vi "reprGraphical.vi"(8 "error in (no error)":errorcluster, 9 "Image Descriptor":T1={"Upper-Left Corner Coordinates"={"UTM Zone"=0, "Hemisphere"=enum."North", "East"=0.0, "North"=0.0}, "Meters/Pixel"=42.294203} {"Upper-Left Corner Coordinates"."North" format="%#_10f"; "Upper-Left Corner Coordinates"."East" format="%#_8f"}, 10 "Image In":T3, 11 "GenericMission in":refnum<class "GenericMission.lvclass">) -> (0 "error out":errorcluster, 2 "Image Out":T3, 3 "GenericMission out":refnum<class "GenericMission.lvclass">)   [LabVIEW 2011, in "GenericMission.lvclass"]
uses:
  GenericMission.lvclass
  <vilib>/vision/Image Controls.llb/IMAQ Image.ctl
  0-OCU/0 Code/mission input/0-Image Descriptor.ctl
  2 Typedefs/UTM Location.ctl
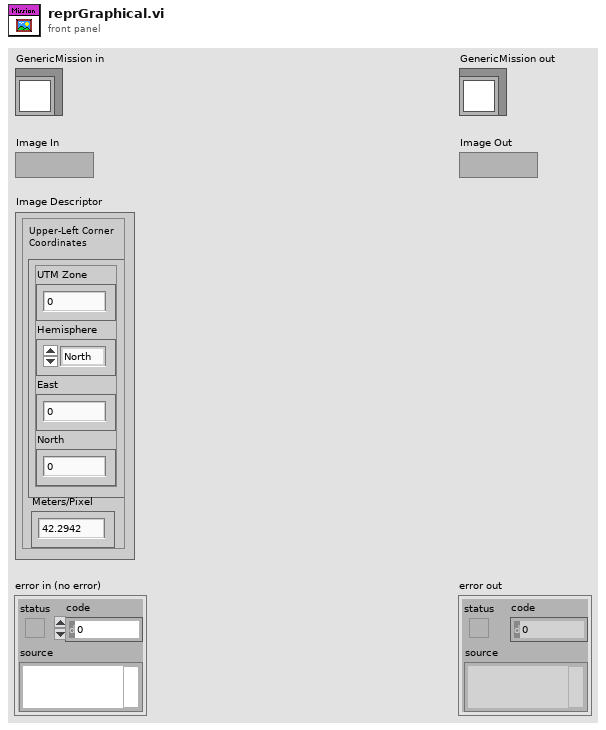
[diagram p1: front panel]
types:
  T1 = typedef "0-Image Descriptor.ctl" = cluster{"Upper-Left Corner Coordinates":T2, "Meters/Pixel":dbl}
  T2 = typedef "UTM Location.ctl" = cluster{"UTM Zone":i32, "Hemisphere":enum16{"North", "South"}, "East":dbl, "North":dbl}
  T3 = typedef "IMAQ Image.ctl" = refnum<image>
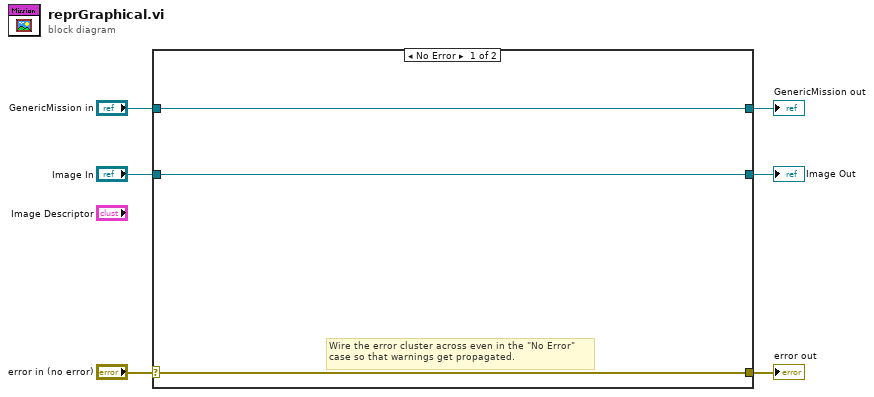
[diagram p0: block diagram]
diagram:
  n1 = case shown="No Error" "error in (no error)" {
    selector: "error in (no error)" -> [w8 w12]
    tunnel: [w8 w12] -> w5
    tunnel: [w9 w11] -> w3
    tunnel: "GenericMission in" -> [w9 w11]
    tunnel: "Image In" -> [w7 w10]
    tunnel: [w7 w10] -> w1
    frame No Error {
      # "Wire the error cluster across even in the \"No Error\"\ncase so that warnings get propagated."
    }
    frame Error {
    }
  }
  "error out" <- w5
  "GenericMission out" <- w3
  "Image Out" <- w1
